vi "DataFinder_ExecuteQuery.vi"() -> ()   [LabVIEW 2023]
doc: "This example shows you how to use the DataFinder to search for specific properties of your measurement data. The example first uses the \"Get Indexed Properties\" VI to determine all the indexed text properties, additionally it uses the \"Get Indexed Value List\" VI to provide a list of indexed values for the specified property. The example uses the VIs \"Create Query\" and \"Execute Query\" to create and execute the queries, and displays the search results as text.\n\nRun the example, search in several properties with several values, and click the stop button to exit."
uses:
  <vilib>/DataFinder/DataTypes/object type.ctl
  <vilib>/DataFinder/DataTypes/operator.ctl
  <vilib>/userdefined/High Color/DFDataFinder.ctl
  <vilib>/DataFinder/DataTypes/property.ctl
  <vilib>/DataFinder/DataTypes/data type.ctl
  <vilib>/DataFinder/Create Query (String).vi
  <vilib>/DataFinder/Close Reference (Results).vi
  <vilib>/DataFinder/Close Reference (Query).vi
  <vilib>/DataFinder/Close Reference (DataFinder).vi
  <vilib>/DataFinder/NI_DataFinder.lvlib
  <vilib>/userdefined/NI_DataFinder Controls.lvlib
panel:
  in  "DataFinder":T1
  in  "Stop Button":bool
  in  "GetValueList":bool
  out "channel properties":string[](array[string])
  out "group properties":string[](array[string])
  out "file properties":string[](array[string])
  in  "Object Type":T2 items=["File", "Channel Group", "Channel"]
  in  "Property Name":string(combo)="fileName"
  in  "Value":string="TR_*"
  out "Results Count":i32
  out "Fullpaths":path[](array[path])
  out "Channel Group Names":string[](array[string])
  out "Channel Names":string[](array[string])
  in  "Search for":T2 items=["File", "Channel Group", "Channel"]
  in  "Search":bool
  in  "Operator":T3 items=["AND", "OR"]
  out "DataPlugin Names":string[](array[string])
  # "Overview: Executes a query using a registered DataFinder.\nRequirements: Select a registered DataFinder which has indexed the TDM Server Demo Data.\nInstructions:\n1. Ensure that the selected DataFinder is already running.\n2. To use the predefined search values ensure the folder [all users]\\Documents\\National Instruments\\DataFinder or one of its parent folders is included in your search areas.\n3. Run the VI.\n4. Choose from the list of indexed string properties in which property the DataFinder is to search for the value you specify. \n5. Specify whether you want to receive the complete resulting files or only the resulting channel groups or channels and click the Search button.\n6. View the identification information for the search results.  \n7. Click Stop to stop the VI."
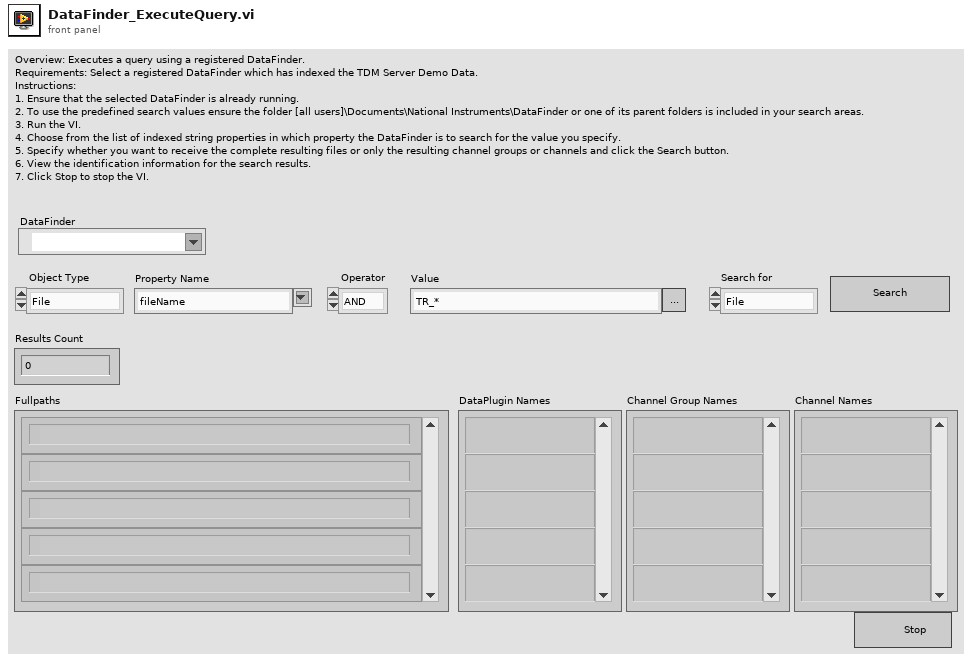
[diagram p1: front panel]
types:
  T1 = typedef "NI_DataFinder Controls.lvlib/DFDataFinder.ctl" = refnum<k21>
  T2 = typedef "NI_DataFinder.lvlib/object type.ctl" = u16
  T3 = typedef "NI_DataFinder.lvlib/operator.ctl" = u16
  T4 = typedef "NI_DataFinder.lvlib/property.ctl" = cluster{"object type":T2, "property name":string, "data type":T5}
  T5 = typedef "NI_DataFinder.lvlib/data type.ctl" = u16
  T6 = typedef "NI_DataFinder Controls.lvlib/DFQuery.ctl" = refnum<k20>
  T7 = typedef "NI_DataFinder Controls.lvlib/DFSearchResult.ctl" = refnum<k20>
  T8 = typedef "NI_DataFinder.lvlib/results elements.ctl" = cluster{"fullpaths":path[], "DataPlugin names":string[], "channel group names":string[], "channel names":string[]}
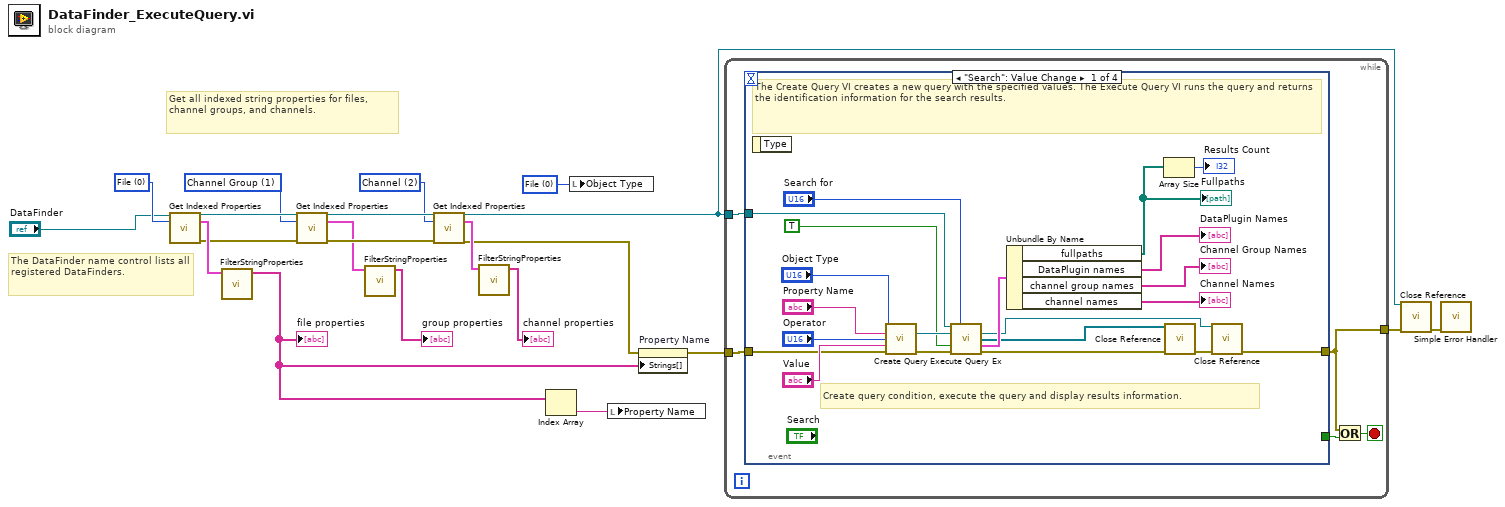
[diagram p0: block diagram]
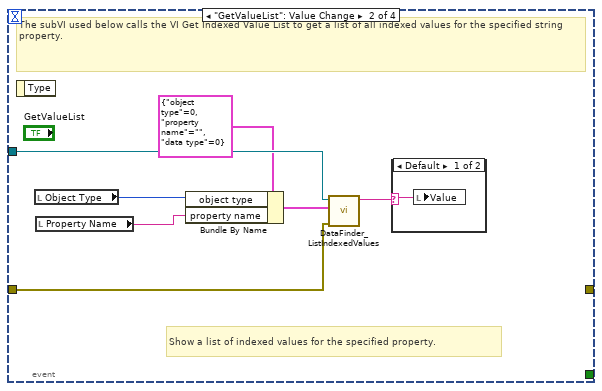
[diagram p2: hidden frame]
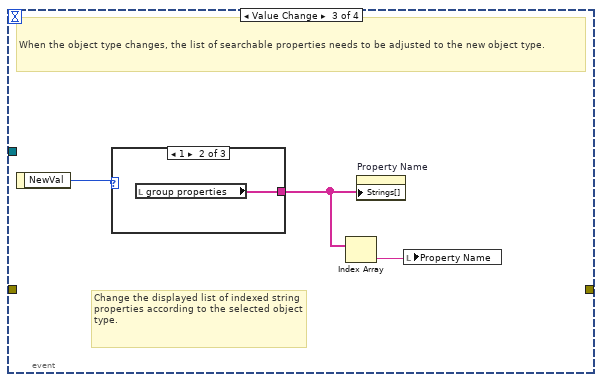
[diagram p4: hidden frame]
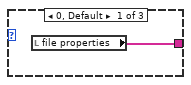
[diagram p5: hidden frame]
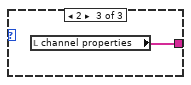
[diagram p6: hidden frame]
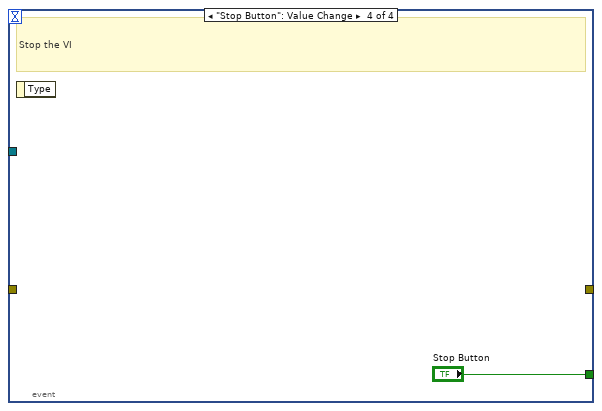
[diagram p7: hidden frame]
diagram:
  w8 = T2 2 items=["File", "Channel Group", "Channel"] ("object type")
  w9 = T2 1 items=["File", "Channel Group", "Channel"] ("object type")
  w10 = T2 0 items=["File", "Channel Group", "Channel"] ("object type")
  w5 = u16 0 items=["File", "Channel Group", "Channel"]
  # "The DataFinder name control lists all registered DataFinders."
  # "Get all indexed string properties for files, channel groups, and channels."
  n1 = call <vilib>:"Get Indexed Properties.vi"("DataFinder reference"="DataFinder", "object type"=w10) -> ("DataFinder reference out"=w17:T1, "properties"=w21:T4[], "error out"=w18:errorcluster)  [unwired: 11 in]
  n2 = call "FilterStringProperties.vi"("properties"=w21) -> ("string properties"=w19:string[])  [unwired: 10 in]
  "file properties" <- w19
  n3 = call <vilib>:"Get Indexed Properties.vi"("DataFinder reference"=w17, "object type"=w9, "error in (no error)"=w18) -> ("DataFinder reference out"=w16:T1, "properties"=w14:T4[], "error out"=w15:errorcluster)  [unwired: 10 in]
  n4 = call "FilterStringProperties.vi"("properties"=w14) -> ("string properties"=→"group properties":string[])  [unwired: 10 in]
  n5 = call <vilib>:"Get Indexed Properties.vi"("DataFinder reference"=w16, "object type"=w8, "error in (no error)"=w15) -> ("DataFinder reference out"=w2:T1, "properties"=w12:T4[], "error out"=w4:errorcluster)  [unwired: 10 in]
  n6 = call "FilterStringProperties.vi"("properties"=w12) -> ("string properties"=→"channel properties":string[])  [unwired: 10 in]
  n7 = Index Array(array=w19) -> (element=w3:string)  [unwired: 1 in]
  n8 = local write "Object Type"(w5) -> ()
  n9 = local write "Property Name"(w3) -> ()
  n10 = property on="Property Name" class="CmbBox"(error in=w4, "Strings[]"=w19) -> (error out=w20:errorcluster)  [unwired: 1 in, 1 out]
  n11 = while {
    tunnel: w2 -> [w25]
    tunnel: w20 -> [w26]
    tunnel: [w22] -> w1
    stop <- w23 stop-if-true
    n12 = event shown="[0] \"Search\": Value Change" {
      selector: _ -> [_ _ _ _]
      dyn-events: _ -> [_ _ _ _]
      timeout: _ -> [_ _ _ _]
      tunnel: w25 -> [w35 w54 _ _]
      tunnel: w26 -> [w33 w53 _ _]
      tunnel: [_ _ _ "Stop Button"] -> w24
      tunnel: [w28 _ _ _] -> w22
      event "Search": Value Change {
        # "Create query condition, execute the query and display results information."
        # "The Create Query VI creates a new query with the specified values. The Execute Query VI runs the query and returns the identification information for the search results."
        n13 = event-data() -> ()  [unwired: 2 out]
        n14 = call-poly <vilib>:"Create Query.vi"("object type"="Object Type", "property name"="Property Name", "comparison operator (=)"="Operator", "value"="Value", "error in (no error)"=w33) -> ("query reference out"=w40:T6, "error out"=w45:errorcluster)  [unwired: 9 in]
        n15 = call <vilib>:"Execute Query Ex.vi"("DataFinder reference"=w35, "result object type (file)"="Search for", "query reference"=w40, "fill results elements? (F)"=TRUE, "error in (no error)"=w45) -> ("query reference out"=w29:T6, "result references out"=w31:T7[], "results elements"=w41:T8, "error out"=w30:errorcluster)  [unwired: 5 in, 2 out]
        n16 = Unbundle By Name(w41) -> ("fullpaths"=w42:path[], "DataPlugin names"=→"DataPlugin Names":string[], "channel group names"=→"Channel Group Names":string[], "channel names"=→"Channel Names":string[])
        "Fullpaths" <- w42
        n17 = Array Size(array=w42) -> (size(s)=→"Results Count":i32)
        n18 = call-poly <vilib>:"Close Reference.vi"("result references"=w31, "error in (no error)"=w30) -> ("error out"=w32:errorcluster)  [unwired: 13 in]
        n19 = call-poly <vilib>:"Close Reference.vi"("query reference"=w29, "error in (no error)"=w32) -> ("error out"=w28:errorcluster)  [unwired: 13 in]
      }
      event "GetValueList": Value Change {
        # "Show a list of indexed values for the specified property."
        # "The subVI used below calls the VI Get Indexed Value List to get a list of all indexed values for the specified string property."
        n20 = event-data() -> ()  [unwired: 2 out]
        n21 = local read "Object Type"() -> (w50:T2)
        n22 = local read "Property Name"() -> (w48:string)
        n23 = Bundle By Name(cluster=T4 {"object type"=0, "property name"="", "data type"=0} ("property"), "object type"=w50, "property name"=w48) -> (w51:T4)
        n24 = call "DataFinder_ListIndexedValues.vi"("error in (no error)"=w53, "property"=w51, "DataFinder"=w54) -> ("Value"=w49:string)  [unwired: 8 in]
        n25 = case shown="Default" w49 {
          selector: w49 -> [w55 _]
          frame Default {
            n26 = local write "Value"(w55) -> ()
          }
          frame "" {
          }
        }
      }
      event Value Change {
        # "Change the displayed list of indexed string properties according to the selected object type."
        # "When the object type changes, the list of searchable properties needs to be adjusted to the new object type."
        n27 = event-data() -> ("NewVal"=w58:T2)  [unwired: 1 out]
        n28 = case shown="1" w58 {
          tunnel: [w59 w60 w61] -> w57
          frame 0, Default {
            n29 = local read "file properties"() -> (w59:string[])
          }
          frame 1 {
            n30 = local read "group properties"() -> (w60:string[])
          }
          frame 2 {
            n31 = local read "channel properties"() -> (w61:string[])
          }
        }
        n32 = Index Array(array=w57) -> (element=w56:string)  [unwired: 1 in]
        n33 = property on="Property Name" class="CmbBox"("Strings[]"=w57) -> ()  [unwired: 2 in, 2 out]
        n34 = local write "Property Name"(w56) -> ()
      }
      event "Stop Button": Value Change {
        # "Stop the VI"
        n35 = event-data() -> ()  [unwired: 2 out]
      }
    }
    n36 = Or(x=w22, y=w24) -> (x .or. y?=w23:bool)
  }
  n37 = call-poly <vilib>:"Close Reference.vi"("DataFinder reference"=w2, "error in (no error)"=w1) -> ("error out"=w6:errorcluster)  [unwired: 13 in]
  n38 = call <vilib>:"Simple Error Handler.vi"("error in (no error)"=w6) -> ()  [unwired: 2 in, 7 out]
